vi "ReadBitDepth.vi"(8 "error in":errorcluster, 11 "Image Reference In":T1) -> (0 "error out":errorcluster, 2 "BitDepth":u32, 3 "Image Reference Out":T1)   [LabVIEW 2020, in "OpenLvVision_Image.lvlib" / "Management.lvlib"]
doc: "Retruns number of bits per pixel, determining the range of representable colors or shades."
uses:
  Management.lvlib
  TypeDef/Image.ctl
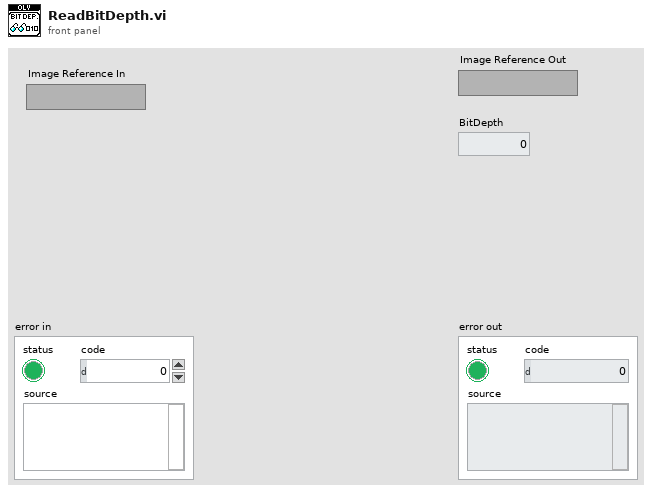
[diagram p1: front panel]
types:
  T1 = typedef "OpenLvVision_Image.lvlib/Management.lvlib/Image.ctl" = refnum<image>
  T2 = typedef "IMAQ Image.ctl" = refnum<image>
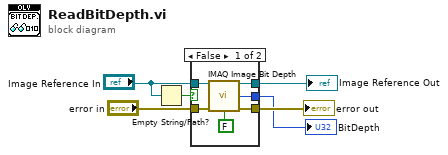
[diagram p0: block diagram]
diagram:
  n1 = Empty String/Path?(string/path="Image Reference In") -> (empty?=w1:bool)
  n2 = case shown="False" w1 {
    tunnel: "error in" -> [w12 w13]
    tunnel: [w11 w13] -> w5
    tunnel: [w10 w14] -> w4
    tunnel: [w9 _] -> w3
    tunnel: "Image Reference In" -> [w8 w14]
    frame False {
      n3 = call "IMAQ Image Bit Depth"("Image"=w8, "error in (no error)"=w12, "Get/Set Bit Depth? (Set)"=FALSE) -> ("Image Out"=w10:T2, "Bit Depth"=w9:u32, "error out"=w11:errorcluster)  [unwired: 10 in]
    }
    frame True {
    }
  }
  "error out" <- w5
  "Image Reference Out" <- w4
  "BitDepth" <- w3
